vi "GetToolsMenuItems.vi"(0 "reference in":refnum<class "Graph.lvclass">, 5 "error in (no error)":errorcluster) -> (14 "reference out":refnum<class "Graph.lvclass">, 16 "ToolMenuItems":T1(array[cluster])=[{"Generate code from UML...", "createScript", "short cut out"={"include Shift key?"=FALSE, "include Ctrl key? "=FALSE, "shortcut key"=""}}, {"Reverse Engineering...", "Class Reversed Engineering", "short cut out"={"include Shift key?"=FALSE, "include Ctrl key? "=TRUE, "shortcut key"="R"}}, {"Auto Place...", "AutoPlace", "short cut out"={"include Shift key?"=FALSE, "include Ctrl key? "=FALSE, "shortcut key"=""}}, {"Synchronize all classes from code", "Synchronize All", "short cut out"={"include Shift key?"=FALSE, "include Ctrl key? "=FALSE, "shortcut key"=""}}, {"Try to straighten associations", "StraightenAssociations", "short cut out"={"include Shift key?"=FALSE, "include Ctrl key? "=TRUE, "shortcut key"="A"}}, {"Toggle auto synchronization", "ToggleSync", "short cut out"={"include Shift key?"=FALSE, "include Ctrl key? "=FALSE, "shortcut key"="F5"}}, {"-", "APP_SEPARATOR", "short cut out"={"include Shift key?"=FALSE, "include Ctrl key? "=FALSE, "shortcut key"=""}}], 19 "error out":errorcluster)   [LabVIEW 2020, in "Graph.lvclass"]
uses:
  <resource>/Framework/Providers/Open_GDS/UML/Graph_class/Graph.lvclass
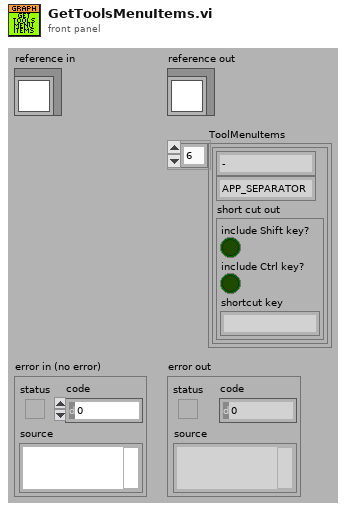
[diagram p1: front panel]
types:
  T1 = cluster{string, string, "short cut out":cluster{"include Shift key?":bool, "include Ctrl key? ":bool, "shortcut key":string}}[]
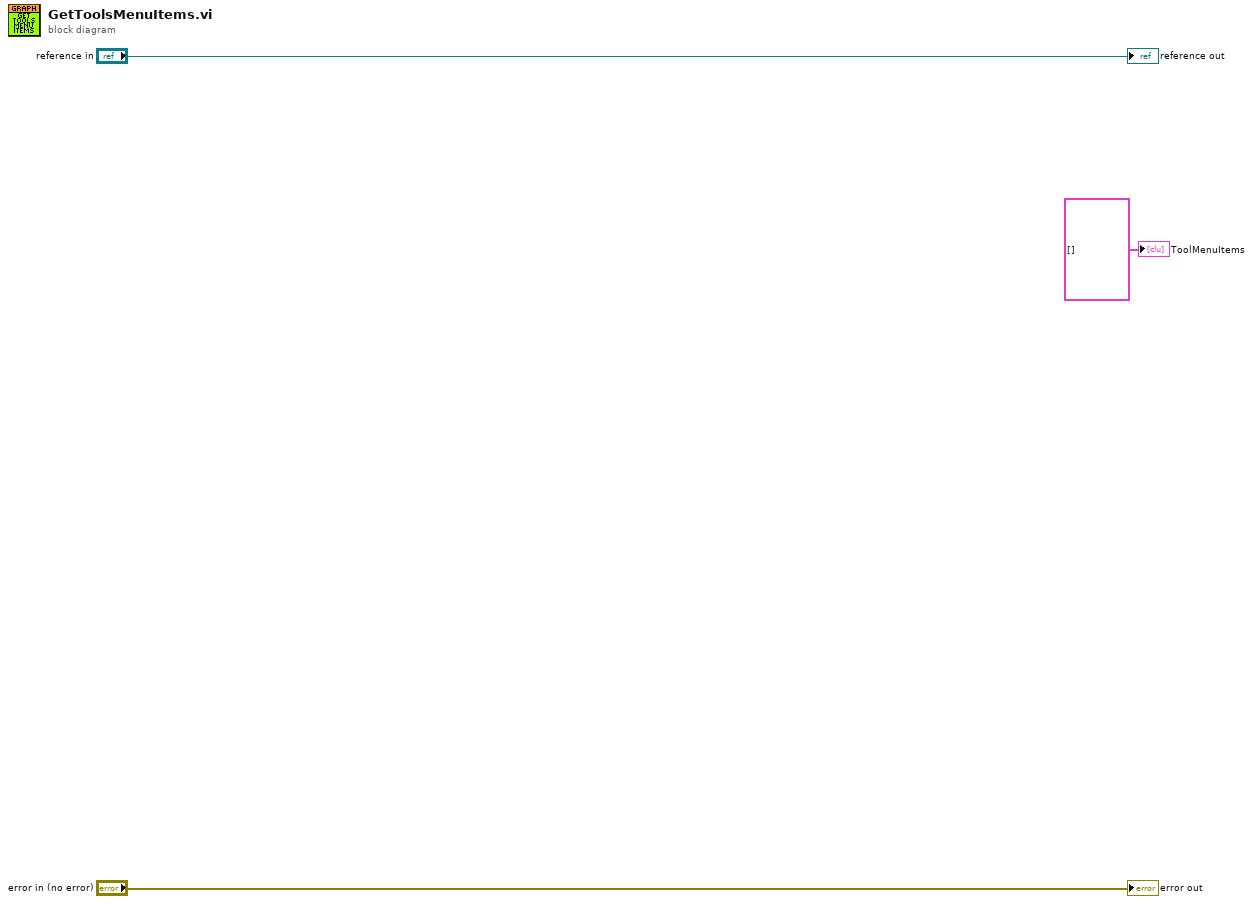
[diagram p0: block diagram]
diagram:
  "error out" <- "error in (no error)"
  "reference out" <- "reference in"
  "ToolMenuItems" <- T1 [] ("ToolMenuItems")
